vi "DS4Monitor.GetDPadInput.vi"(1 "direction info":T2) -> (0 "D-Pad Input":T1)   [LabVIEW 2024]
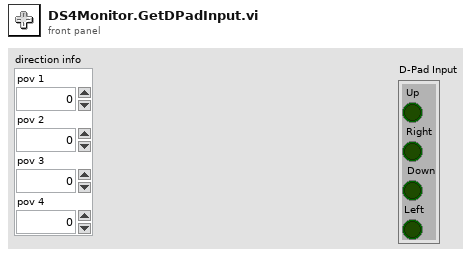
[diagram p1: front panel]
types:
  T1 = cluster{"Up":bool, "Right":bool, "Down":bool, "Left":bool}
  T2 = cluster{"pov 1":i32, "pov 2":i32, "pov 3":i32, "pov 4":i32}
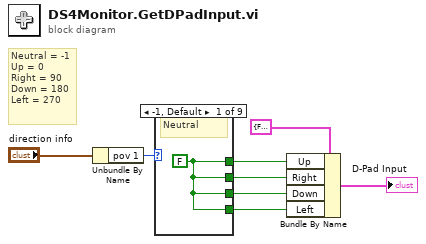
[diagram p0: block diagram]
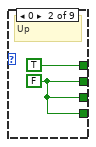
[diagram p2: hidden frame]
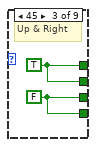
[diagram p3: hidden frame]
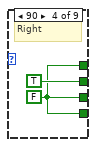
[diagram p4: hidden frame]
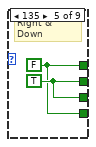
[diagram p5: hidden frame]
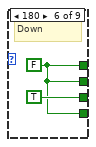
[diagram p6: hidden frame]
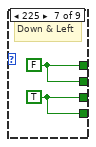
[diagram p7: hidden frame]
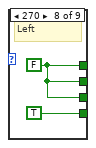
[diagram p8: hidden frame]
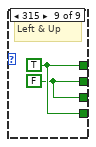
[diagram p9: hidden frame]
diagram:
  # "Neutral = -1\nUp = 0\nRight = 90\nDown = 180\nLeft = 270"
  n1 = Unbundle By Name("direction info") -> ("pov 1"=w5:i32)
  n2 = case shown="-1, Default" w5 {
    tunnel: [w9 TRUE w13 w14 w16 w18 w20 w22 w25] -> w4
    tunnel: [w9 w10 w13 TRUE w17 w18 w20 w22 w24] -> w3
    tunnel: [w9 w10 w12 w14 w17 TRUE w21 w22 w24] -> w2
    tunnel: [w9 w10 w12 w14 w16 w18 w21 TRUE w25] -> w1
    frame -1, Default {
      w9 = FALSE
      # "Neutral"
    }
    frame 0 {
      w10 = FALSE
      # "Up"
    }
    frame 45 {
      w12 = FALSE
      w13 = TRUE
      # "Up & Right"
    }
    frame 90 {
      w14 = FALSE
      # "Right"
    }
    frame 135 {
      w16 = FALSE
      w17 = TRUE
      # "Right & Down"
    }
    frame 180 {
      w18 = FALSE
      # "Down"
    }
    frame 225 {
      w20 = FALSE
      w21 = TRUE
      # "Down & Left"
    }
    frame 270 {
      w22 = FALSE
      # "Left"
    }
    frame 315 {
      w24 = FALSE
      w25 = TRUE
      # "Left & Up"
    }
  }
  n3 = Bundle By Name(cluster=T1 {"Up"=FALSE, "Right"=FALSE, "Down"=FALSE, "Left"=FALSE} ("D-Pad Input"), "Up"=w4, "Right"=w3, "Down"=w2, "Left"=w1) -> (→"D-Pad Input":T1)
